vi "PH_Stepmotor_BaseClass.Evt Call Set Actual Position in Units.vi"(0 "i ref in":refnum<vi>, 1 "Address":T1={"Instance"="N/A", "Motor Nr"=0}, 4 "Position to set [Units]":dbl, 5 "error in":errorcluster) -> (14 "i ref out":refnum<vi>, 19 "error out":errorcluster)   [LabVIEW 2014, in "PH_Stepmotor_BaseClass.lvlib"]
uses:
  PH_Stepmotor_BaseClass.lvlib
  PH_Stepmotor_BaseClass.Axis Address.ctl
  CSCore/CSSystem/CoreLib/CoreLib.double 2 byte array.vi
  CSCore/CSSystem/CoreLib/CoreLib.int 2 byte array.vi
  CSCore/CSSystem/CoreLib/CoreLib.lvlib
  CSCore/BaseProcess/BaseProcess.lvlib
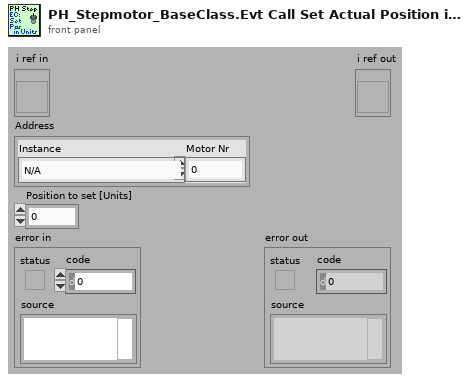
[diagram p1: front panel]
types:
  T1 = typedef "PH_Stepmotor_BaseClass.lvlib/PH_Stepmotor_BaseClass.Axis Address.ctl" = cluster{"Instance":string, "Motor Nr":i32}
  T2 = typedef "CoreDefs.rawDataType.ctl" = i8[]
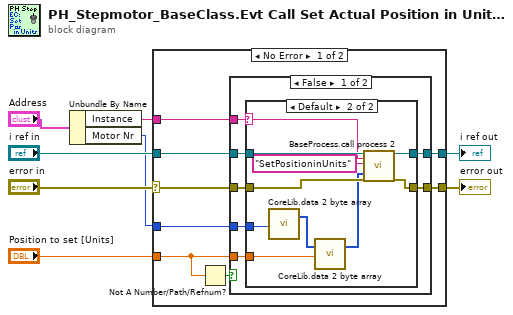
[diagram p0: block diagram]
diagram:
  n1 = Unbundle By Name("Address") -> ("Instance"=w2:string, "Motor Nr"=w1:i32)
  n2 = case shown="No Error" "error in" {
    selector: "error in" -> [w12 w38]
    tunnel: [w16 w38] -> w5
    tunnel: w2 -> [w11 _]
    tunnel: "i ref in" -> [w15 w39]
    tunnel: [w14 w39] -> w7
    tunnel: w1 -> [w13 _]
    tunnel: "Position to set [Units]" -> [w10 _]
    frame No Error {
      n3 = Not A Number/Path/Refnum?(number/path/refnum=w10) -> (NaN/Path/Refnum?=w9:bool)
      n4 = case shown="False" w9 {
        tunnel: [w23 w36] -> w16
        tunnel: w15 -> [w22 w37]
        tunnel: [w21 w37] -> w14
        tunnel: w13 -> [w20 _]
        tunnel: w12 -> [w19 w36]
        tunnel: w11 -> [w18 _]
        tunnel: w10 -> [w17 _]
        frame False {
          n5 = case shown="Default" w18 {
            selector: w18 -> [_ w26]
            tunnel: [w25 w35] -> w23
            tunnel: w19 -> [w25 w33]
            tunnel: w22 -> [w24 w32]
            tunnel: [w24 w31] -> w21
            tunnel: w20 -> [_ w30]
            tunnel: w17 -> [_ w28]
            frame "N/A" {
            }
            frame Default {
              n6 = call-poly "CoreLib.data 2 byte array.vi"("i32"=w30) -> ("byteArray out"=w29:T2)  [unwired: 18 in]
              n7 = call-poly "CoreLib.data 2 byte array.vi"("byteArray"=w29, "f64"=w28) -> ("byteArray out"=w27:T2)  [unwired: 17 in]
              n8 = call "BaseProcess.call process 2.vi"("i ref in"=w32, "Object"=w26, "Selector"="SetPositioninUnits", "Data"=w27, "error in (no error)"=w33) -> ("i ref out"=w31:refnum<vi>, "error out"=w35:errorcluster)  [unwired: 13 in]
            }
          }
        }
        frame True {
        }
      }
    }
    frame Error {
    }
  }
  "i ref out" <- w7
  "error out" <- w5
